vi "Lift Global.vi"() -> ()   [LabVIEW 2018]
panel:
  out "Zero the Lift":bool
  in  "Offset":dbl
  in  "Requested Zone":T1(ring)
  in  "Hatch Panel Auto Height":dbl=9.0
  in  "Hatch Panel 1 Height":dbl=25.5
  in  "Hatch Panel 3 Height":dbl=100.0
  in  "Hatch Panel 2 Height":dbl=66.0
  in  "Cargo Ship Height":dbl=30.0
  in  "Lift Auto Position":u16(ring) items=["Cargo 1", "Hatch 1", "Cargo 2", "Hatch 2", "Cargo 3", "Hatch 3"]
  out "Requested Height":dbl=-0.01886111111111111
  in  "Height PID":T2={"proportional gain (Kc)"=0.06, "integral time(Ti, min)"=0.0, "derivative time(Td, min) 2"=0.001}
  in  "Disable the VI":bool
  out "Current Lift Height":dbl=-0.01886111111111111
  in  "Cargo Zone 3 Height":dbl=94.0
  in  "Cargo Zone 2 Height":dbl=58.0
  in  "Cargo Zone 1 Height":dbl=15.0
  out "Holding current position":bool
  out "Moving to position":bool
  in  "LiftHeight":dbl
  in  "Joystick manual":dbl
  in  "LiftMode":T3(ring)
  in  "LiftMotorSpeedDown":dbl
  in  "LiftLocation":T4(ring)=enum."Cargo Zone 1"
  in  "LiftMotorSpeedUp":dbl
  out "LowerLimit":bool
  out "UpperLimit":bool
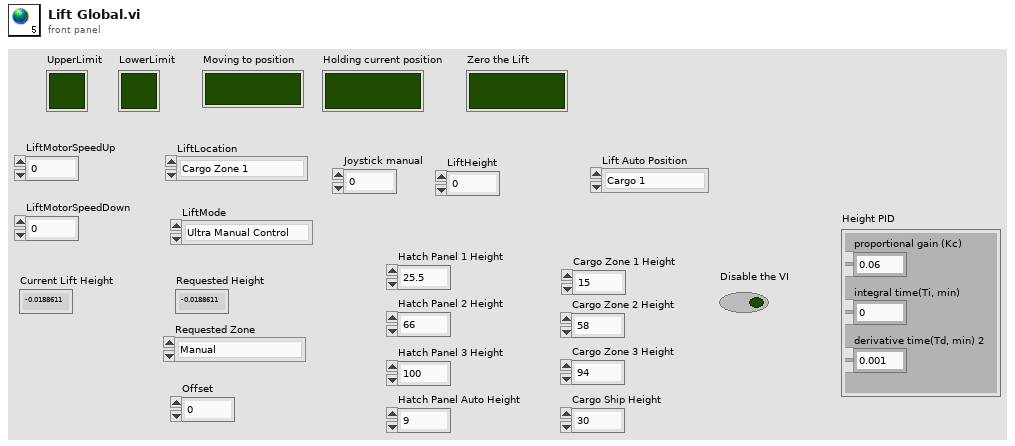
[diagram p1: front panel]
types:
  T1 = enum16{"Manual", "Hatch Panel Zone 1", "Hatch Panel Zone 2", "Hatch Panel Zone 3", "Cargo Zone 1", "Cargo Zone 2", "Cargo Zone 3", "Cargo Ship Zone"}
  T2 = cluster{"proportional gain (Kc)":dbl, "integral time(Ti, min)":dbl, "derivative time(Td, min) 2":dbl}
  T3 = enum16{"Ultra Manual Control", "Manual Control", "Basic Control", "Automated Control", "Autonomous Control"}
  T4 = enum16{"Hatch Panel Zone 1", "Hatch Panel Zone 2", "Hatch Panel Zone 3", "Cargo Zone 1", "Cargo Zone 2", "Cargo Zone 3", "Cargo Ship Zone"}
diagram:
